vi "REPORT_OPRTN_hide_filtered_columns.vi"(9 "ItemNames_in":string[][](array[string]), 10 "hidden_columns":i32[](array[numeric]), 11 "column_headers_in":string[](array[string])) -> (2 "ItemNames_out":string[][](array[string]), 3 "column_headers_out":string[](array[string]))   [LabVIEW 2019]
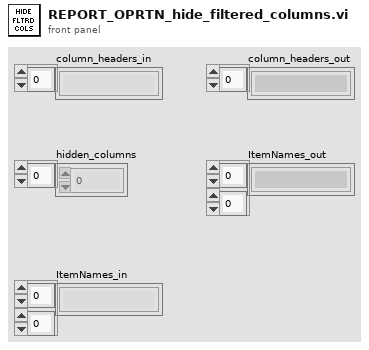
[diagram p1: front panel]
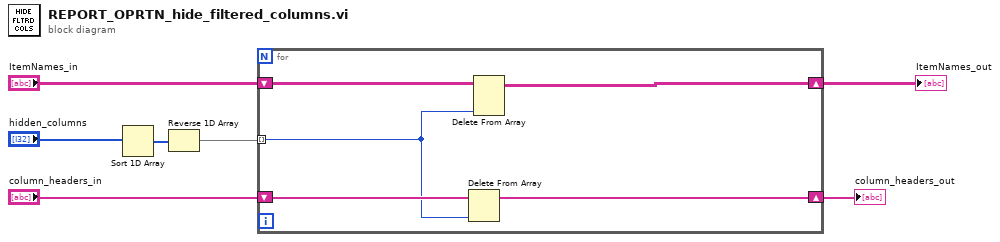
[diagram p0: block diagram]
diagram:
  n1 = Sort 1D Array(array="hidden_columns") -> (sorted array=w2:i32[])
  n2 = Reverse 1D Array(array=w2) -> (reversed array=w1:i32[])
  n3 = for {
    tunnel: w1 -> [w8] mode=indexing
    shift-right: [w9] -> w7
    shift-left: "column_headers_in" -> [w10]
    shift-right: [w11] -> w6
    shift-left: "ItemNames_in" -> [w12]
    n4 = Delete From Array(array=w10, index=w8) -> (array with subset deleted=w9:string[])  [unwired: 1 in, 1 out]
    n5 = Delete From Array(array=w12, index (col)=w8) -> (array with subset deleted=w11:string[][])  [unwired: 2 in, 1 out]
  }
  "column_headers_out" <- w7
  "ItemNames_out" <- w6
